vi "ChangeRightSubpanel.vi"(8 "error in (no error)":errorcluster, 10 "Left Active":i32, 11 "MAUI in":refnum<class "MAUI.lvclass">) -> (0 "error out":errorcluster, 3 "MAUI out":refnum<class "MAUI.lvclass">)   [LabVIEW 2016, in "MAUI.lvclass"]
uses:
  MAUI.lvclass
  MAUI.lvclass/MAUI.ctl
  <vilib>/Levylab/Embedded SMO UI/EmbeddedSMO.lvclass
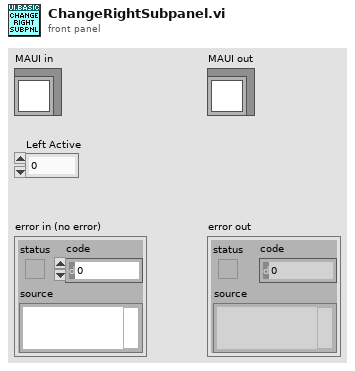
[diagram p1: front panel]
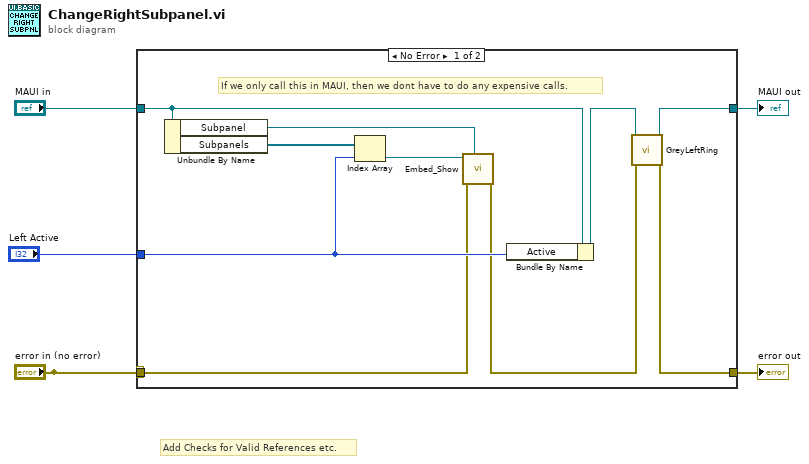
[diagram p0: block diagram]
diagram:
  # "Add Checks for Valid References etc."
  n1 = case shown="No Error" "error in (no error)" {
    selector: "error in (no error)" -> [_ w17]
    tunnel: [w6 w17] -> w5
    tunnel: [w8 w16] -> w3
    tunnel: "MAUI in" -> [w11 w16]
    tunnel: "Left Active" -> [w15 _]
    tunnel: "error in (no error)" -> [w10 _]
    frame No Error {
      # "If we only call this in MAUI, then we dont have to do any expensive calls."
      n2 = Unbundle By Name(w11) -> ("Subpanel"=w14:refnum<vi>, "Subpanels"=w13:refnum<class "EmbeddedSMO.lvclass">[])
      n3 = Index Array(array=w13, index=w15) -> (element=w12:refnum<class "EmbeddedSMO.lvclass">)
      n4 = call <vilib>:"Embed_Show.vi"("Sub Panel"=w14, "error in (no error)"=w10, "EmbeddedSMO in"=w12) -> ("error out"=w7:errorcluster)  [unwired: 7 in, 1 out]
      n5 = Bundle By Name(cluster=w11, "Active"=w15) -> (w9:refnum<class "MAUI.lvclass">)
      n6 = call "GreyLeftRing.vi"("error in (no error)"=w7, "MAUI in"=w9) -> ("error out"=w6:errorcluster, "MAUI out"=w8:refnum<class "MAUI.lvclass">)  [unwired: 8 in]
    }
    frame Error {
    }
  }
  "error out" <- w5
  "MAUI out" <- w3
